vi "open images.vi"() -> ()   [LabVIEW 2009]
uses:
  <vilib>/picture/picture.llb/imagedata.ctl
panel:
  out "progress":u8(slide) scale=0.0..841.0
  out "image data":cluster{"name":string[], "image data":T1[]}
  out "files opened":string[](array[string])
  in  "abort":bool
  out "curently opening":string
  out "files not yet opened":path[](array[path])
  out "unopenable files":path[](array[path])
  in  "Path":path
  # "only allows PNGs, BMPs, and JPEGs"
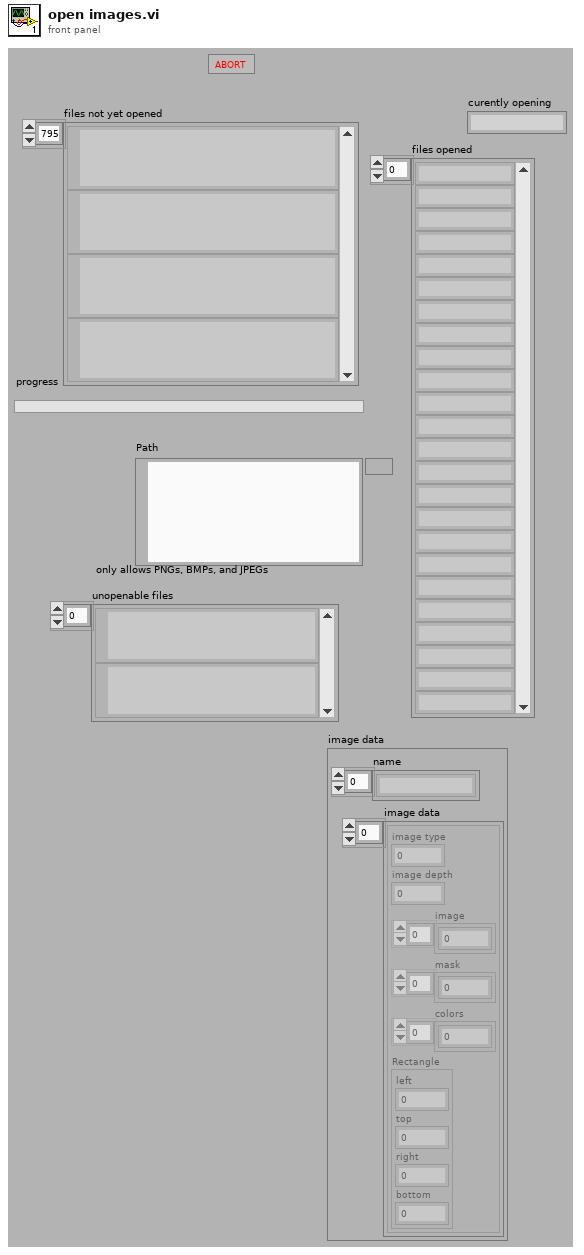
[diagram p1: front panel]
types:
  T1 = typedef "imagedata.ctl" = cluster{"image type":i32, "image depth":i32, "image":u8[], "mask":u8[], "colors":u32[], "Rectangle":cluster{"left":i16, "top":i16, "right":i16, "bottom":i16}}
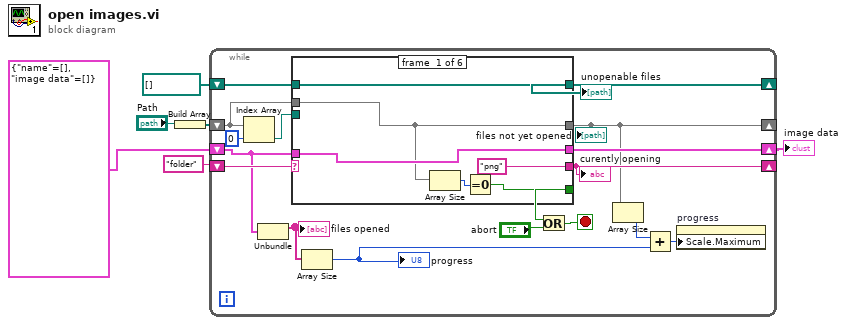
[diagram p0: block diagram]
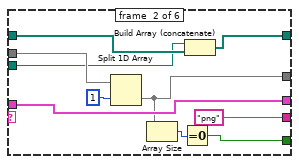
[diagram p2: hidden frame]
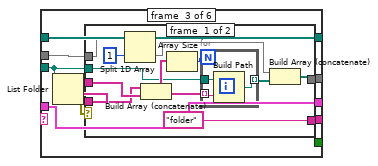
[diagram p3: hidden frame]
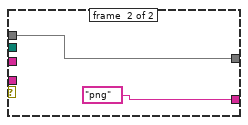
[diagram p4: hidden frame]
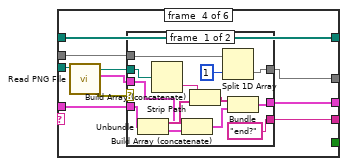
[diagram p5: hidden frame]
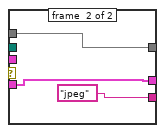
[diagram p6: hidden frame]
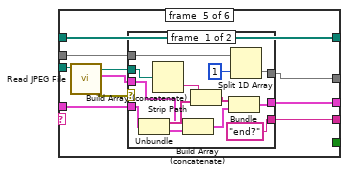
[diagram p7: hidden frame]
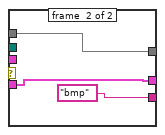
[diagram p8: hidden frame]
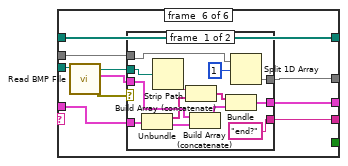
[diagram p9: hidden frame]
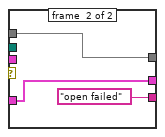
[diagram p10: hidden frame]
diagram:
  n1 = Build Array("Path") -> (w5:path[])
  n2 = while {
    shift-right: [w20] -> _
    shift-left: "folder" -> [w23]
    shift-right: [w10] -> _
    shift-left: w5 -> [w19]
    shift-right: [w17] -> _
    shift-left: path[] [] -> [w18]
    shift-right: [w16] -> w1
    shift-left: cluster{"name":string[], "image data":T1[]} {"name"=[], "image data"=[]} ("Cluster") -> [w15]
    stop <- w13 stop-if-true
    n3 = Index Array(array=w19, index=0) -> (element=w22:path)
    n4 = Unbundle(w15) -> ("name"=w11:string[])  [unwired: 1 out]
    "files opened" <- w11
    n5 = case shown="\"folder\"" w23 {
      tunnel: [w24 w34 w46 w68 w94 w120] -> w10
      tunnel: w22 -> [_ w30 w45 w73 w99 w125]
      tunnel: ["png" "png" w43 w71 w97 w123] -> w20
      tunnel: w19 -> [w24 w39 w42 w70 w96 w122]
      tunnel: w18 -> [w25 w31 w41 w69 w95 w121]
      tunnel: [w25 w36 w41 w69 w95 w121] -> w17
      tunnel: [w28 w35 w40 w66 w92 w117] -> w16
      tunnel: w15 -> [w28 w35 w40 w65 w91 w118]
      tunnel: [w26 w32 _ _ _ _] -> w12
      frame #0 {
        n6 = Array Size(array=w24) -> (size(s)=w27:i32)
        n7 = Equal To 0?(x=w27) -> (x = 0?=w26:bool)
      }
      frame #1 {
        n8 = Split 1D Array(array=w39, index=1) -> (second subarray=w34:path[])  [unwired: 1 out]
        n9 = Array Size(array=w34) -> (size(s)=w33:i32)
        n10 = Equal To 0?(x=w33) -> (x = 0?=w32:bool)
        n11 = Build Array (concatenate)(w30, w31) -> (w36:path[])
      }
      frame #2 {
        n12 = List Folder(path=w45) -> (filenames=w48:string[], folder names=w47:string[], error out=w44:errorcluster)  [unwired: 3 in, 1 out]
        n13 = case shown="No Error" w44 {
          tunnel: w48 -> [w56 _]
          tunnel: w47 -> [w55 _]
          tunnel: [w52 w63] -> w46
          tunnel: w45 -> [w57 _]
          tunnel: ["folder" "png"] -> w43
          tunnel: w42 -> [w51 w63]
          frame #0 {
            n14 = Split 1D Array(array=w51, index=1) -> (second subarray=w50:path[])  [unwired: 1 out]
            n15 = Build Array (concatenate)(w55, w56) -> (w58:string[])
            n16 = Array Size(array=w58) -> (size(s)=w59:i32)
            n17 = for {
              N: w59 -> [_]
              tunnel: w58 -> [w62] mode=indexing
              tunnel: w57 -> [w61]
              tunnel: [w60] -> w53 mode=indexing
              n18 = Build Path(base path=w61, name or relative path=w62) -> (appended path=w60:path)
            }
            n19 = Build Array (concatenate)(w50, w53) -> (w52:path[])
          }
          frame #1 {
          }
        }
      }
      frame #3 {
        n20 = call <vilib>:"Read PNG File.vi"("path to PNG file"=w73) -> ("error out"=w72:errorcluster, "image data"=w74:T1, "path"=w67:path)  [unwired: 8 in]
        n21 = case shown="No Error" w72 {
          tunnel: w74 -> [w78 _]
          tunnel: ["end?" "jpeg"] -> w71
          tunnel: w70 -> [w77 w89]
          tunnel: [w76 w89] -> w68
          tunnel: w67 -> [w86 _]
          tunnel: [w85 w88] -> w66
          tunnel: w65 -> [w81 w88]
          frame #0 {
            n22 = Unbundle(w81) -> ("name"=w80:string[], "image data"=w79:T1[])
            n23 = Strip Path(path=w86) -> (name=w83:string)  [unwired: 1 out]
            n24 = Build Array (concatenate)(w78, w79) -> (w82:T1[])
            n25 = Build Array (concatenate)(w83, w80) -> (w84:string[])
            n26 = Split 1D Array(array=w77, index=1) -> (second subarray=w76:path[])  [unwired: 1 out]
            n27 = Bundle(w84, w82) -> (w85:cluster{string[], T1[]})  [unwired: 1 in]
          }
          frame #1 {
          }
        }
      }
      frame #4 {
        n28 = call <vilib>:"Read JPEG File.vi"("path to JPEG file"=w99) -> ("error out"=w98:errorcluster, "image data"=w100:T1, "path"=w93:path)  [unwired: 8 in]
        n29 = case shown="No Error" w98 {
          tunnel: w100 -> [w104 _]
          tunnel: ["end?" "bmp"] -> w97
          tunnel: w96 -> [w102 w115]
          tunnel: [w103 w115] -> w94
          tunnel: w93 -> [w112 _]
          tunnel: [w111 w114] -> w92
          tunnel: w91 -> [w107 w114]
          frame #0 {
            n30 = Unbundle(w107) -> ("name"=w106:string[], "image data"=w105:T1[])
            n31 = Strip Path(path=w112) -> (name=w109:string)  [unwired: 1 out]
            n32 = Build Array (concatenate)(w104, w105) -> (w108:T1[])
            n33 = Build Array (concatenate)(w109, w106) -> (w110:string[])
            n34 = Bundle(w110, w108) -> (w111:cluster{string[], T1[]})  [unwired: 1 in]
            n35 = Split 1D Array(array=w102, index=1) -> (second subarray=w103:path[])  [unwired: 1 out]
          }
          frame #1 {
          }
        }
      }
      frame #5 {
        n36 = call <vilib>:"Read BMP File.vi"("path to BMP file"=w125) -> ("error out"=w124:errorcluster, "image data"=w126:T1, "path"=w119:path)  [unwired: 8 in]
        n37 = case shown="No Error" w124 {
          tunnel: w126 -> [w137 _]
          tunnel: ["end?" "open failed"] -> w123
          tunnel: w122 -> [w129 w141]
          tunnel: [w128 w141] -> w120
          tunnel: w119 -> [w138 _]
          tunnel: [w130 w140] -> w117
          tunnel: w118 -> [w131 w140]
          frame #0 {
            n38 = Unbundle(w131) -> ("name"=w133:string[], "image data"=w132:T1[])
            n39 = Strip Path(path=w138) -> (name=w134:string)  [unwired: 1 out]
            n40 = Build Array (concatenate)(w134, w133) -> (w135:string[])
            n41 = Build Array (concatenate)(w137, w132) -> (w136:T1[])
            n42 = Bundle(w135, w136) -> (w130:cluster{string[], T1[]})  [unwired: 1 in]
            n43 = Split 1D Array(array=w129, index=1) -> (second subarray=w128:path[])  [unwired: 1 out]
          }
          frame #1 {
          }
        }
      }
    }
    "unopenable files" <- w17
    "files not yet opened" <- w10
    "curently opening" <- w20
    n44 = Array Size(array=w11) -> (size(s)=w8:i32)
    "progress" <- w8
    n45 = Or(x=w12, y="abort") -> (x .or. y?=w13:bool)
    n46 = Array Size(array=w10) -> (size(s)=w9:i32)
    n47 = Add(x=w9, y=w8) -> (x+y=w7:i32)
    n48 = property on="progress" class="Slide (strict)"("Scale.Maximum"=w7) -> ()  [unwired: 2 in, 2 out]
  }
  "image data" <- w1
